vi "Package Must Exist.vi"(8 "error in (no error)":errorcluster, 11 "InstallAction in":refnum<class "InstallAction.lvclass">) -> (0 "error out":errorcluster, 2 "Pkg Must Exist":bool, 3 "InstallAction out":refnum<class "InstallAction.lvclass">)   [LabVIEW 2020, in "GPackTools.lvlib" / "InstallAction.lvclass"]
uses:
  InstallAction.lvclass
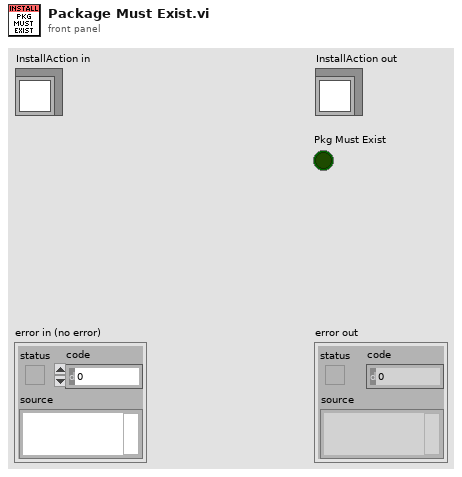
[diagram p1: front panel]
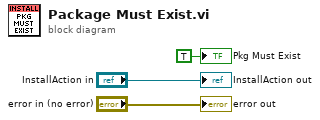
[diagram p0: block diagram]
diagram:
  "error out" <- "error in (no error)"
  "InstallAction out" <- "InstallAction in"
  "Pkg Must Exist" <- TRUE ("Pkg Must Exist")
